vi "H5Fopen_mod.vi"(8 "error in (no error)":errorcluster, 9 "fcpl_id":T1 format="%.0x", 10 "mode (read-only)":T2, 11 "path":path) -> (0 "error out":errorcluster, 1 "file exists?":bool, 3 "ref out":T1 format="%.0x")   [LabVIEW 2018]
doc: "Open the specified path as an HDF5 file. Mode specifies how the file should be opened and what to do if it does/doesn't exist.\n\nWhen creating files, a File Creation Property List (fcpl) can be specified with <b>fcpl_id</b> to configure advanced settings."
uses:
  <vilib>/addons/h5labview2/base/hid_t.ctl
  <vilib>/addons/h5labview2/file/H5Fmode.ctl
  <vilib>/addons/h5labview2/file/H5F.lvlib
panel:
  out "path out":path
  # "h5labview :: H5Fopen"
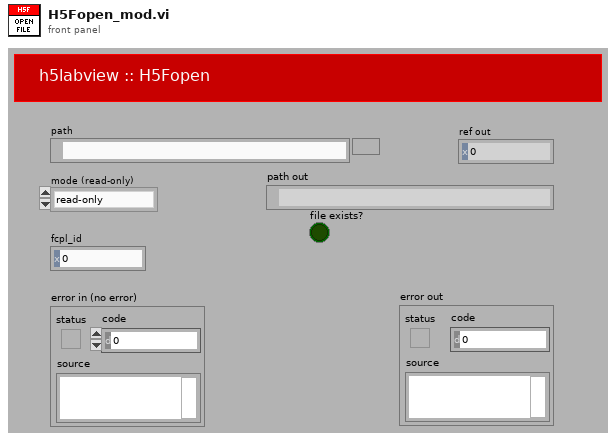
[diagram p1: front panel]
types:
  T1 = typedef "hid_t.ctl" = i32
  T2 = typedef "H5F.lvlib/H5Fmode.ctl" = enum16{"read-only", "read-write", "overwrite", "create new", "open or create"}
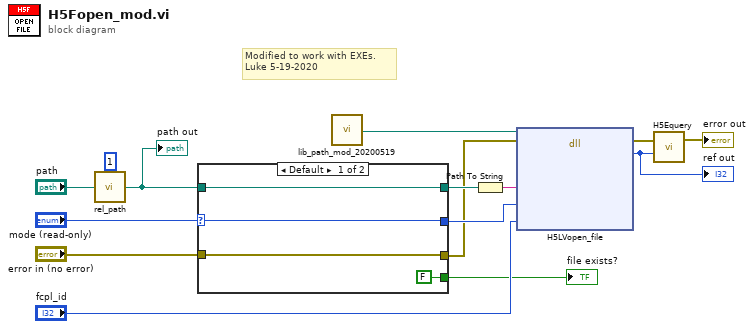
[diagram p0: block diagram]
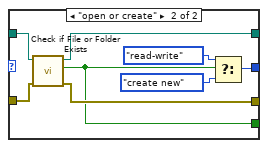
[diagram p2: hidden frame]
diagram:
  # "Modified to work with EXEs. \nLuke 5-19-2020"
  n1 = call <vilib>:"rel_path.vi"("rel path"="path", "bump"=u8 1 ("steps")) -> ("path"=w8:path)
  "path out" <- w8
  n2 = case shown="Default" "mode (read-only)" {
    selector: "mode (read-only)" -> [w19 _]
    tunnel: [w19 w25] -> w9
    tunnel: w8 -> [w18 w24]
    tunnel: [w17 w23] -> w4
    tunnel: [w18 w22] -> w5
    tunnel: "error in (no error)" -> [w17 w21]
    tunnel: [FALSE ("file or folder exists?") w20] -> w2
    frame Default {
    }
    frame "open or create" {
      n3 = call <vilib>:"Check if File or Folder Exists.vi"("error in (no error)"=w21, "path"=w24) -> ("error out"=w23:errorcluster, "file or folder exists?"=w20:bool, "dup path"=w22:path)  [unwired: 7 in]
      n4 = Select(t=H5Fmode."read-write" ("mode"), s=w20, f=H5Fmode."create new" ("mode")) -> (s? t:f=w25:T2)
    }
  }
  "file exists?" <- w2
  n5 = call "lib_path_mod_20200519.vi"() -> ("path"=w1:path)  [unwired: 2 in]
  n6 = Path To String(path=w5) -> (string=w11:string)
  n7 = dll-call lib="?" fn="H5LVopen_file"(path in=w1, error in=w4, "name"=w11, "flags"=w9, "fpcl_id"="fcpl_id") -> (error out=w10:errorcluster, "return type"=w13:i32)  [unwired: 6 in, 1 out]
  "ref out" <- w13
  n8 = call <vilib>:"H5Equery.vi"("retval"=w13, "error in (no error)"=w10) -> ("error out"=→"error out":errorcluster)  [unwired: 1 in]
